vi "request.vi"(7 "LabVIEW Web Service Request":refnum<class "Web Request.lvclass">) -> ()   [LabVIEW 2017]
uses:
  <vilib>/wsapi/Web Request.lvclass
  <vilib>/NI/NI JSONRPC Server Framework/Classes/Server/Send Request (Sync).vi
panel:
  # "Use the Web Service Request input terminal to call the VIs on the Web Services palette. Do not remove it from the connector pane unless you don't need access to the palette."
  # "Each additional control wired to the connector pane will be available as an input in the URL. To include an indicator in terminal-mode output (the default setting), it must also be wired to the connector pane."
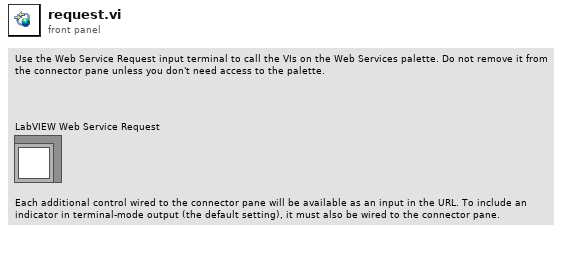
[diagram p1: front panel]
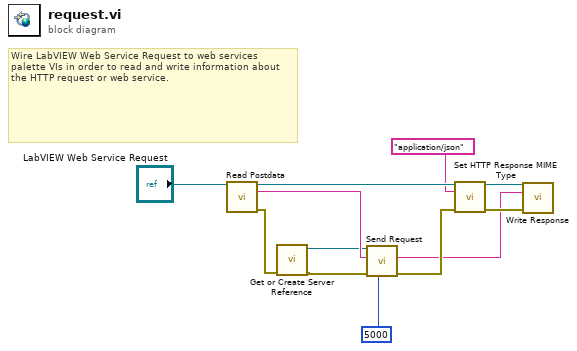
[diagram p0: block diagram]
diagram:
  # "Wire LabVIEW Web Service Request to web services palette VIs in order to read and write information about the HTTP request or web service."
  n1 = call <vilib>:"Read Postdata.vi"("LabVIEW Web Service Request"="LabVIEW Web Service Request") -> ("LabVIEW Web Service Request out"=w6:refnum<class "Web Request.lvclass">, "postdata"=w11:string, "error out"=w2:errorcluster)  [unwired: 12 in]
  n2 = call <vilib>:"Get or Create Server Reference.vi"("error in (no error)"=w2) -> ("error out"=w3:errorcluster, "Server Out"=w4:refnum<class "JSONRPC Server.lvclass">)  [unwired: 9 in]
  n3 = call-poly <vilib>:"Send Request.vi"("Timeout (-1)"=5000, "error in (no error)"=w3, "JSON Request String"=w11, "JSONRPC Server in"=w4) -> ("error out"=w8:errorcluster, "JSON Response String"=w7:string)  [unwired: 5 in, 1 out]
  n4 = call <vilib>:"Set HTTP Response MIME Type.vi"("LabVIEW Web Service Request"=w6, "MIME type (text/html)"="application/json" ("header"), "error in (no error)"=w8) -> ("LabVIEW Web Service Request out"=w10:refnum<class "Web Request.lvclass">, "error out"=w9:errorcluster)  [unwired: 11 in]
  n5 = call <vilib>:"Write Response.vi"("LabVIEW Web Service Request"=w10, "response string"=w7, "error in (no error)"=w9) -> ()  [unwired: 11 in, 2 out]
